vi "Control Mode Read Single.vi"(8 "error in":errorcluster, 9 "Channel Index":i32, 11 "Cycler in":refnum<class "Cycler.lvclass">) -> (0 "error out":errorcluster, 1 "Changed or First Call?":bool, 2 "Control Mode CTL":u16, 3 "Cycler out":refnum<class "Cycler.lvclass">)   [LabVIEW 2023, in "Cycler.lvclass"]
uses:
  Cycler.lvclass
  Cycler.lvclass/Cycler.ctl
  Low Level Capabilities/Control Mode/Control Mode.lvclass
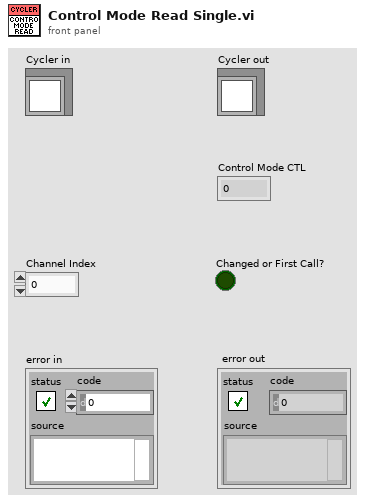
[diagram p1: front panel]
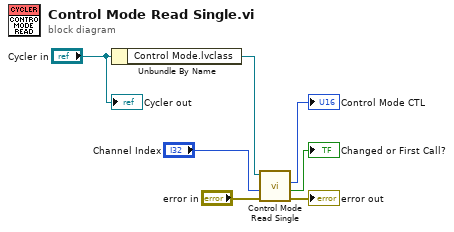
[diagram p0: block diagram]
diagram:
  n1 = Unbundle By Name("Cycler in") -> ("Control Mode.lvclass"=w2:refnum<class "Control Mode.lvclass">)
  n2 = call-dynamic "Control Mode Read Single.vi"("error in"="error in", "Channel Index"="Channel Index", "Control Mode in"=w2) -> ("error out"=→"error out":errorcluster, "Changed or First Call?"=→"Changed or First Call?":bool, "Control Mode CTL"=→"Control Mode CTL":u16)  [unwired: 5 in, 1 out]
  "Cycler out" <- "Cycler in"
